vi "Bernards.vi"() -> ()   [LabVIEW 2018]
uses:
  <userlib>/KE237.LLB/Keith 237 Operate/Standby.vi
  <vilib>/Utility/file.llb/Write Delimited Spreadsheet (string).vi
  <instrlib>/Keithley 24XX/Keithley 24XX.lvlib
  <vilib>/Analysis/NI_AALBase.lvlib
panel:
  out "error 2":string
  out "error":string
  in  "Delay Gate (s) 2":dbl=60.0 format="%#.3g"
  in  "source/measure (V/I:0)":u16(ring)=1 items=["voltage/current", "current/voltage"]
  in  "Setpoint Array":dbl[](array[numeric])=[-2e-08, -5e-08, -1e-07]
  in  "Autozero?":u16(ring)=2 items=["On", "Off", "Once"]
  in  "Measurement Speed (1 PLC)":dbl=1.0 format="%.2g"
  in  "Manual Range (Max I)":dbl=1.0
  in  "Enable Meas Auto Range":bool=TRUE
  in  "Source Mode":u16(ring) items=["Voltage", "Current"]
  in  "Initial Gate Setting":dbl format="%#.3g"
  in  "Voltage Compliance Limit 237 (V)":dbl=-0.95 format="%#.3f"
  in  "Current Compliance\nLimit 237 (A)":fxp<+/-,64,32>=0.10000000009313226
  in  "Delay Gate (s)":dbl=30.0 format="%#.3g"
  in  "Keithley 237 GPIB address":string="17"
  in  "Wait Time Btwn Keithley Readings (ms)":i32=30
  out "Time Btwn Iterations (ms)":i32
  out "Total Elapsed Time (ms)":i32
  out "# Avgs":i32
  out "Current (A)":dbl format="%.2e"
  in  "Total Measure Time (s)":dbl=120.0 format="%#.3g"
  in  "Drain Bias (V)":dbl=-0.6 format="%#.3g"
  in  "Current Compliance\nLimit (A)":dbl=0.5 format="%#.3e"
  in  "Keithley 2400\nVISA resource":refnum<visa-resource-name>="GPIB0::24::INSTR"
  in  "ApproximateTime Step (ms)":dbl=300.0 format="%#.3g"
  in  "Current Offset":dbl format="%^#_3e"
  out "I-t Measurement\nBy M. Ziffer 7/3/2014":cluster{dbl[], dbl[]}(graph)={[-2.0, -1.95, -1.9, -1.85, -1.8, -1.75, -1.7, -1.65, -1.6, -1.55, -1.5, -1.45, -1.4, -1.35, -1.2999999999999998, -1.25, -1.2, -1.15, -1.1, -1.0499999999999998, -1.0, -0.95, -0.8999999999999999, -0.8499999999999999, -0.7999999999999998, -0.75, -0.7, -0.6499999999999999, -0.5999999999999999, -0.5499999999999998, -0.5, -0.44999999999999996, -0.3999999999999999, -0.34999999999999987, -0.2999999999999998, -0.25, -0.19999999999999996, -0.1499999999999999, -0.09999999999999987, -0.04999999999999982, 0.0, 0.050000000000000266, 0.10000000000000009, 0.1499999999999999, 0.20000000000000018, 0.25, 0.30000000000000027, 0.3500000000000001, 0.40000000000000036, 0.4500000000000002, 0.5, 0.5500000000000003, 0.6000000000000001, 0.6500000000000004, 0.7000000000000002, 0.75, 0.8000000000000003, 0.8500000000000001, 0.9000000000000004, 0.9500000000000002, 1.0, 1.0500000000000003, 1.1, 1.1500000000000004, 1.2000000000000002, 1.25, 1.3000000000000003, 1.35, 1.4000000000000004, 1.4500000000000002, 1.5, 1.5500000000000003, 1.6, 1.6500000000000004, 1.7000000000000002, 1.75, 1.8000000000000003, 1.85, 1.9000000000000004, 1.9500000000000002, 2.0, 1.95, 1.9, 1.85, 1.8, 1.75, 1.7, 1.65, 1.6, 1.55, 1.5, 1.45, 1.4, 1.35, 1.2999999999999998, 1.25, 1.2, 1.15, 1.1, 1.0499999999999998, 1.0, 0.95, 0.8999999999999999, 0.8499999999999999, 0.7999999999999998, 0.75, 0.7, 0.6499999999999999, 0.5999999999999999, 0.5499999999999998, 0.5, 0.44999999999999996, 0.3999999999999999, 0.34999999999999987, 0.2999999999999998, 0.25, 0.19999999999999996, 0.1499999999999999, 0.09999999999999987, 0.04999999999999982, 0.0, -0.050000000000000266, -0.10000000000000009, -0.1499999999999999, -0.20000000000000018, -0.25, -0.30000000000000027, -0.3500000000000001, -0.40000000000000036, -0.4500000000000002, -0.5, -0.5500000000000003, -0.6000000000000001, -0.6500000000000004, -0.7000000000000002, -0.75, -0.8000000000000003, -0.8500000000000001, -0.9000000000000004, -0.9500000000000002, -1.0, -1.0500000000000003, -1.1, -1.1500000000000004, -1.2000000000000002, -1.25, -1.3000000000000003, -1.35, -1.4000000000000004, -1.4500000000000002, -1.5, -1.5500000000000003, -1.6, -1.6500000000000004, -1.7000000000000002, -1.75, -1.8000000000000003, -1.85, -1.9000000000000004, -1.9500000000000002, -2.0], [-0.9617289445307117, -0.9618513744908972, -0.9601574911889584, -0.9603488957746004, -0.9598860982876659, -0.9595594700613103, -0.9590290885663679, -0.9586886097902229, -0.9580144940757807, -0.9570474587019399, -0.9571418538143588, -0.9562287187728303, -0.9551771894828052, -0.9535572870291384, -0.9535421571112963, -0.9533114258642045, -0.9520938012261039, -0.9513117179729429, -0.9508812384355169, -0.9504840780921618, -0.9504173840793213, -0.9482281628421478, -0.9464640811713977, -0.9453356785488072, -0.9439408336230415, -0.9428695575652444, -0.9416178906119992, -0.9396031084275935, -0.9378375248899987, -0.9354517815949719, -0.9324159524550173, -0.928767917889437, -0.9245502864168607, -0.9203528467096396, -0.9146985405384399, -0.908595454304189, -0.9012966039381313, -0.8917361646028689, -0.8808115851751085, -0.8684870433493713, -0.853007079283089, -0.8360736418594031, -0.8154860511533626, -0.7920970894092216, -0.7641180332150388, -0.7294003786125389, -0.6854183749419586, -0.6263231964633708, -0.5399961516707377, -0.4044042921440459, -0.19129744134883978, 0.11936942255465804, 0.5420583260977958, 1.0996962734707192, 1.8318907919106253, 2.7834859177196174, 3.9948214605959804, 5.494887344369723, 7.293988211209965, 9.39251059714275, 11.765998658717283, 14.371720946722268, 17.153138293174568, 20.070768287470067, 23.082285540692517, 26.15604905590766, 29.26009131920428, 32.38734131897913, 35.54092126952808, 38.70923397757575, 41.89103456238207, 45.09512285116253, 48.318234786641504, 51.57411300669423, 54.84161623237131, 58.130390342544004, 61.4596508891188, 64.79419021952893, 68.17503711098149, 71.57587551887687, 75.0023346626475, 71.8977923333163, 68.72637799211101, 65.51757272894447, 62.2950059155054, 59.076872390492845, 55.84672949319313, 52.615591470047114, 49.383497814590335, 46.15858586388574, 42.93308596012382, 39.714879010509975, 36.494540522470736, 33.276879251143754, 30.087779593472593, 26.903443634933772, 23.758388169345494, 20.669969771208738, 17.671195580039395, 14.804861569698371, 12.12778391916459, 9.68736655227705, 7.528128139792144, 5.673530623057721, 4.128839936603901, 2.8787577310032053, 1.895544581260216, 1.1383875896205915, 0.5622048852612092, 0.12746496878202787, -0.18928305409978952, -0.4042961076690051, -0.5411369085387429, -0.6286316214282486, -0.6871327837574404, -0.7298882072135505, -0.7640718647157413, -0.7921132761963248, -0.8155779431543743, -0.8358809022810104, -0.8523300154596555, -0.8668520109778625, -0.8802307520791266, -0.8907705198464766, -0.8998007445608903, -0.9078572589377096, -0.9150023626386364, -0.9215738644543149, -0.925261336930741, -0.9288795566582202, -0.9332418679701618, -0.9352489739462505, -0.9376688708058178, -0.9394550911063516, -0.9405290371496502, -0.9430050037047499, -0.9440335043698243, -0.9453382929096107, -0.9473152502994113, -0.9474565926568992, -0.9494901203645137, -0.94896546821346, -0.9503187058651598, -0.9511280452203158, -0.9523093469306558, -0.9532668704811476, -0.9541692143312739, -0.9545545822386634, -0.955485183435348, -0.9561708134622656, -0.956805602515258, -0.9577699122788996, -0.9578049002139094, -0.9580356870856992, -0.958780001168953, -0.9592832934359943, -0.9588639388381576, -0.959203916992021, -0.9603773199952523, -0.9611007191920772, -0.9623172869609168]}
  in  "First bias settle (ms)":dbl=2000.0 format="%#.2f"
  out "Outputfile":path
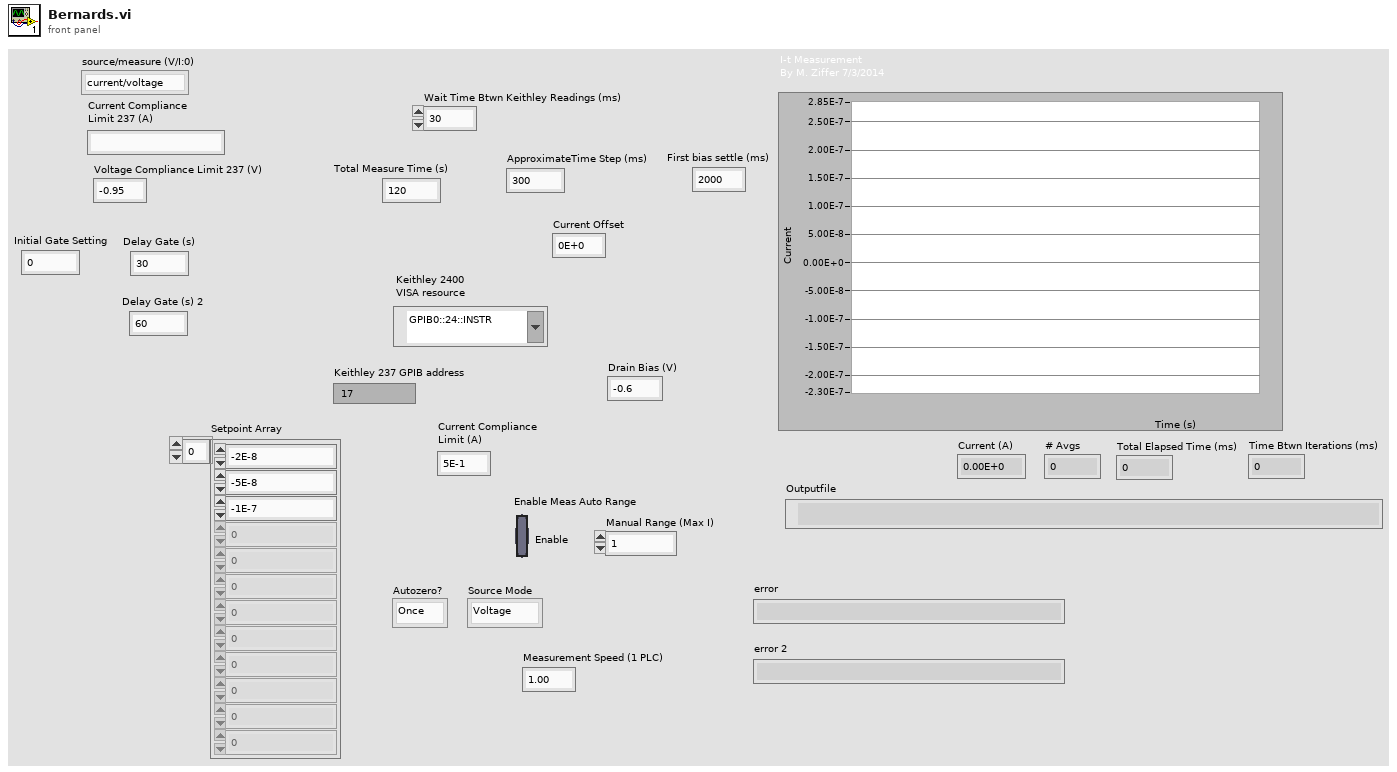
[diagram p1: front panel]
types:
  T1 = cluster{"error":bool, "code":i32, "source":string}
  T2 = cluster{"source value":string, "measure value":string, "delay value (sec)":string, "time value (sec)":string}[]
  T3 = cluster{"source value":dbl, "measure value":dbl, "delay value (sec)":dbl, "time value (sec)":dbl}[]
  T4 = cluster{"[0]":cluster{"source value":dbl, "measure value":dbl, "delay value (sec)":dbl, "time value (sec)":dbl}, "[1]":cluster{"source value":dbl, "measure value":dbl, "delay value (sec)":dbl, "time value (sec)":dbl}, "[2]":cluster{"source value":dbl, "measure value":dbl, "delay value (sec)":dbl, "time value (sec)":dbl}, "[3]":cluster{"source value":dbl, "measure value":dbl, "delay value (sec)":dbl, "time value (sec)":dbl}, "[4]":cluster{"source value":dbl, "measure value":dbl, "delay value (sec)":dbl, "time value (sec)":dbl}, "[5]":cluster{"source value":dbl, "measure value":dbl, "delay value (sec)":dbl, "time value (sec)":dbl}, "[6]":cluster{"source value":dbl, "measure value":dbl, "delay value (sec)":dbl, "time value (sec)":dbl}, "[7]":cluster{"source value":dbl, "measure value":dbl, "delay value (sec)":dbl, "time value (sec)":dbl}, "[8]":cluster{"source value":dbl, "measure value":dbl, "delay value (sec)":dbl, "time value (sec)":dbl}}
  T5 = cluster{"source value":dbl, "measure value":dbl, "delay value (sec)":dbl, "time value (sec)":dbl}
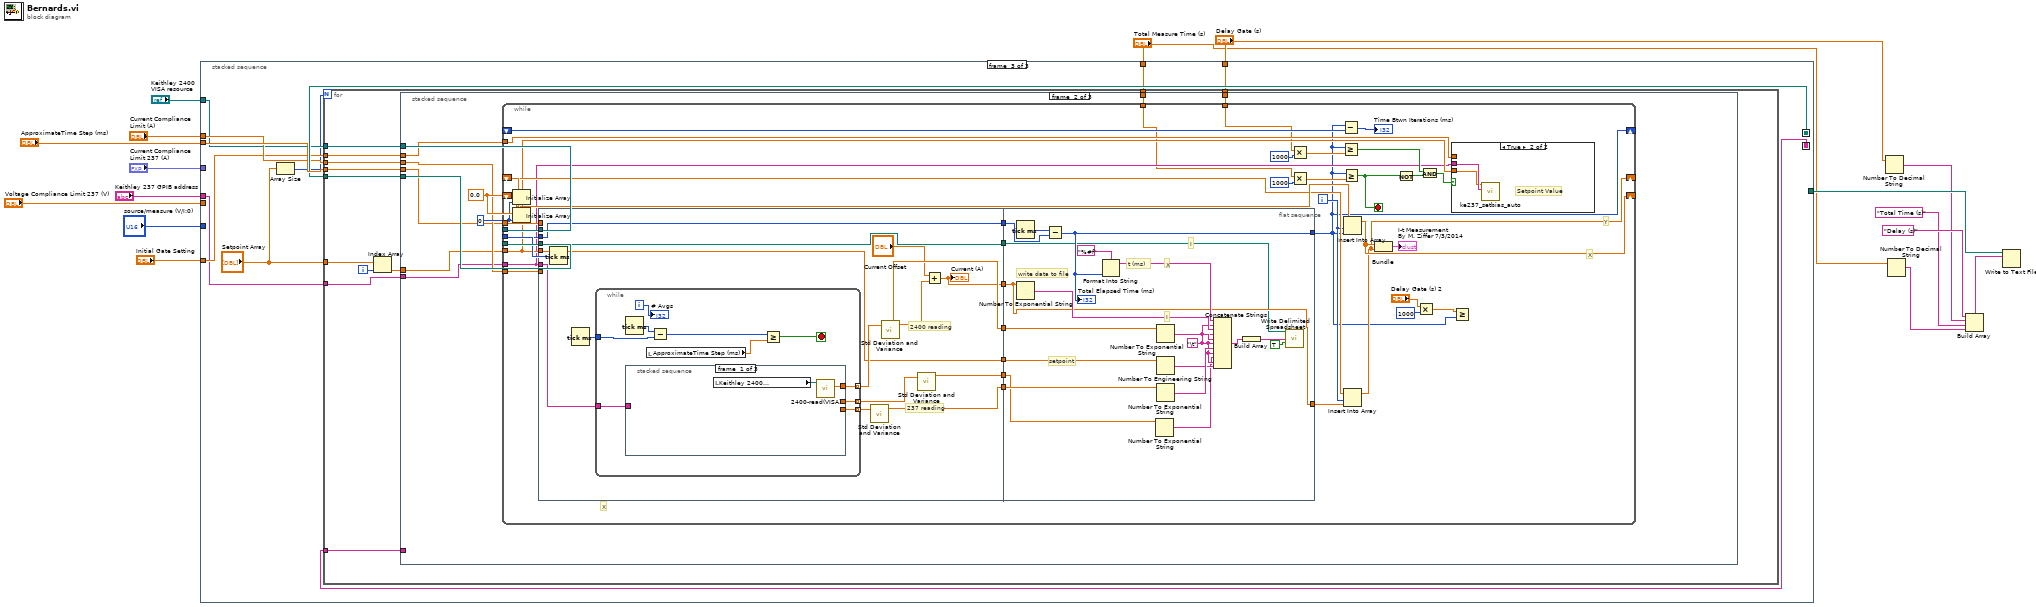
[diagram p0: block diagram]
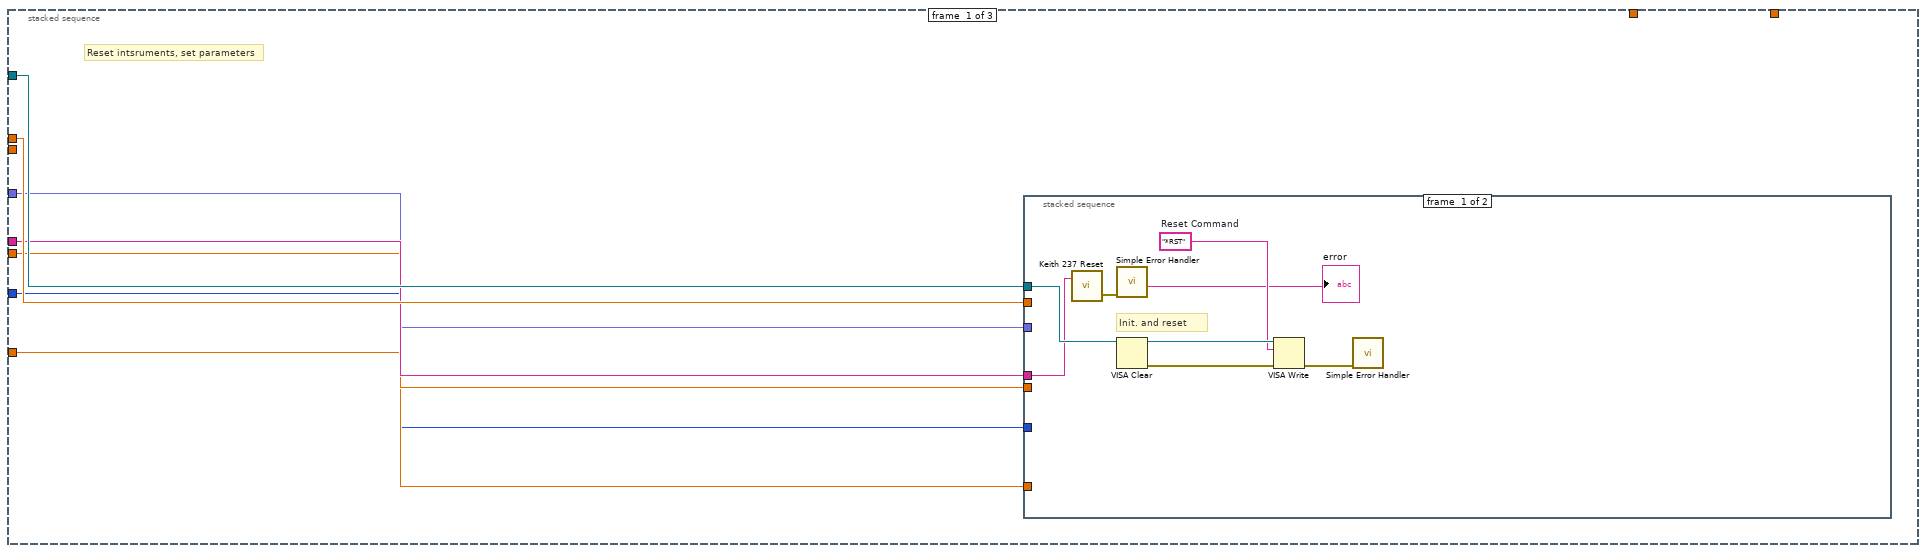
[diagram p2: hidden frame]
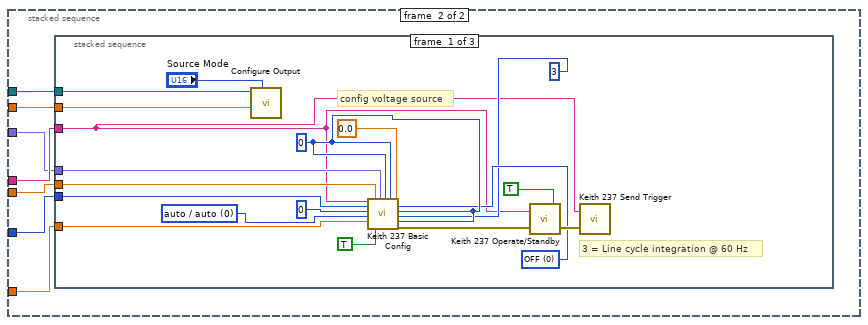
[diagram p3: hidden frame]
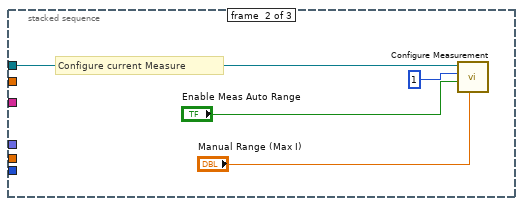
[diagram p4: hidden frame]
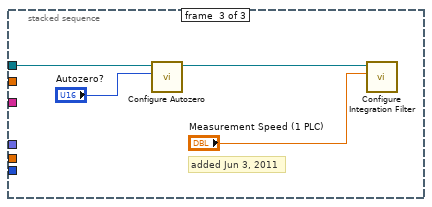
[diagram p5: hidden frame]
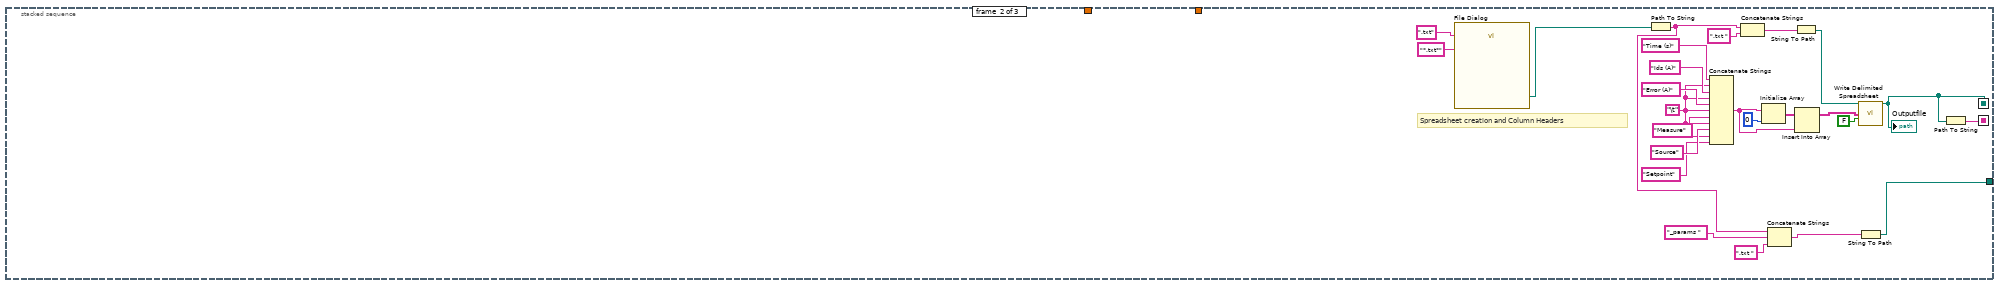
[diagram p6: hidden frame]
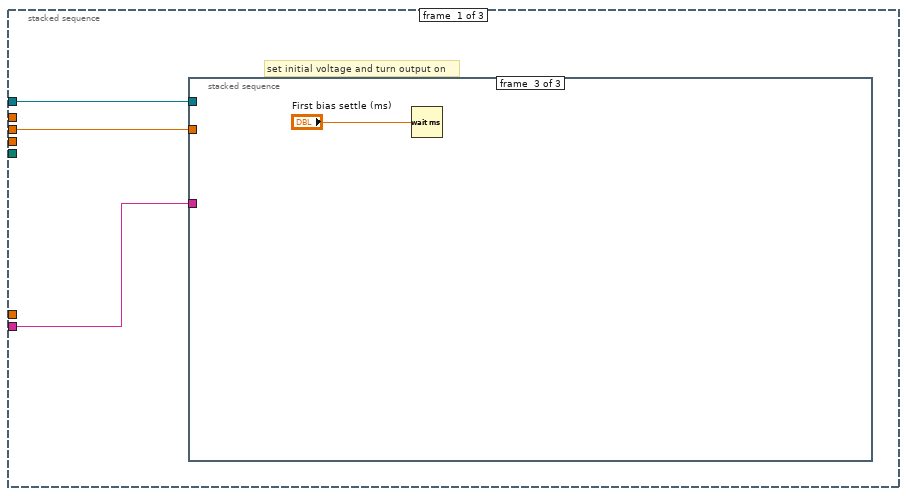
[diagram p7: hidden frame]
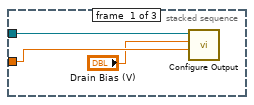
[diagram p8: hidden frame]
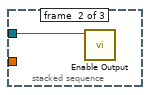
[diagram p9: hidden frame]
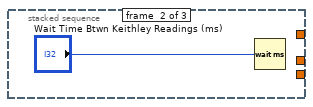
[diagram p10: hidden frame]
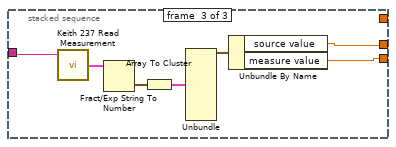
[diagram p11: hidden frame]
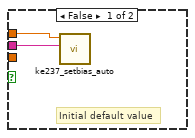
[diagram p12: hidden frame]
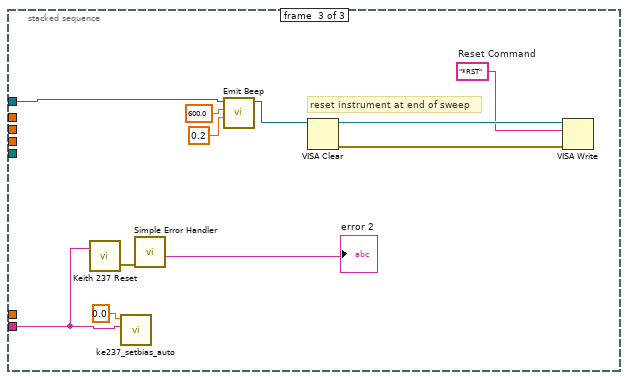
[diagram p13: hidden frame]
diagram:
  n1 = stacked-sequence {
    seq-local: [_ w70 _] -> [_ _ w99]
    seq-local: [_ w89 _] -> [_ _ w98]
    tunnel: "ApproximateTime Step (ms)" -> [_ _ w100]
    tunnel: "Keithley 2400\nVISA resource" -> [w22 _ w96]
    tunnel: "Current Compliance\nLimit (A)" -> [w23 _ w97]
    tunnel: "Keithley 237 GPIB address" -> [w21 _ w94]
    tunnel: "Voltage Compliance Limit 237 (V)" -> [w19 _ _]
    tunnel: "Current Compliance\nLimit 237 (A)" -> [w20 _ _]
    tunnel: "Initial Gate Setting" -> [w18 _ w95]
    tunnel: "source/measure (V/I:0)" -> [w17 _ _]
    tunnel: [_ w65 _] -> w6
    tunnel: "Delay Gate (s)" -> [_ _ w91]
    tunnel: "Total Measure Time (s)" -> [_ _ w90]
    frame #0 {
      # "Reset intsruments, set parameters"
      n2 = stacked-sequence {
        tunnel: w22 -> [w31 w37]
        tunnel: w23 -> [_ w38]
        tunnel: w21 -> [w25 w36]
        tunnel: w20 -> [_ w35]
        tunnel: w19 -> [_ w34]
        tunnel: w18 -> [_ w33]
        tunnel: w17 -> [_ w32]
        frame #0 {
          w29 = "*RST"  # Reset Command
          # "Init. and reset"
          n3 = call <userlib>:"Keith 237 Reset.vi"("GPIB address"=w25) -> ("error out"=w26:T1)  [unwired: 1 in]
          n4 = call <vilib>:"Simple Error Handler.vi"("error in (no error)"=w26) -> ("source out"=→"error":string)  [unwired: 1 in, 7 out]
          n5 = VISA Clear(VISA resource name=w31) -> (VISA resource name out=w30:refnum<visa-resource-name>, error out=w28:errorcluster)  [unwired: 1 in]
          n6 = VISA Write(VISA resource name=w30, write buffer=w29, error in (no error)=w28) -> (error out=w27:errorcluster)  [unwired: 2 out]
          n7 = call <vilib>:"Simple Error Handler.vi"("error in (no error)"=w27) -> ()  [unwired: 1 in, 8 out]
        }
        frame #1 {
          n8 = stacked-sequence {
            tunnel: w37 -> [w56 w59 w63]
            tunnel: w38 -> [w55 _ _]
            tunnel: w36 -> [w40 _ _]
            tunnel: w35 -> [w43 _ _]
            tunnel: w34 -> [w42 _ _]
            tunnel: w33 -> [w41 _ _]
            tunnel: w32 -> [w39 _ _]
            frame #0 {
              w45 = u16 0 items=["OFF", "ON"] ("default delay (on:1)")
              w46 = u16 0 items=["auto / auto", "1 nA / 1.1 V", "10 nA / 11 V", "100 nA / 110 V", "0.001 mA / 1100 V", "0.01 mA / 1100 V", "0.1 mA / 1100 V", "1 mA / 1100 V", "10 mA / 1100 V", "100 mA / 1100 V"] ("source range\nI source / V source (auto:0)")
              w48 = u16 0
              # "3 = Line cycle integration @ 60 Hz"
              # "config voltage source"
              n9 = call <instrlib>:"Configure Output.vi"("Source Mode  (0: Voltage)"="Source Mode", "Compliance  Level (0.1)"=w55, "VISA resource name"=w56) -> ()  [unwired: 3 in, 6 out]
              n10 = call <userlib>:"Keith 237 Basic Config.vi"("GPIB address"=w40, "source/measure (V/I:0)"=w39, "function (DC:0)"=u16 0, "source range\nI source / V source (auto:0)"=w46, "source level"=w41, "voltage \ncompliance level"=w42, "1100 V range (disabled:F)"=TRUE, "current \ncompliance level"=w43, "compliance/\nmeasurement range (auto:0)"=w48, "suppression (off:0)"=w48, "DC delay (sec)"=0.0, "default delay (on:1)"=w45, "filter (disabled:0)"=w48, "integration time (medium:1)"=u16 3, "sense (local:0)"=w48) -> ("error out"=w53:T1)  [unwired: 4 in]
              n11 = call "Keith 237 Operate/Standby.vi"("source"=TRUE, "error in"=w53, "GPIB address"=w40) -> ("error out"=w51:T1)
              n12 = call <userlib>:"Keith 237 Send Trigger.vi"("GPIB address"=w40, "error in"=w51) -> ()  [unwired: 1 out]
            }
            frame #1 {
              # "Configure current Measure"
              n13 = call <instrlib>:"Configure Measurement.vi"("Manual Range (1.0)"="Manual Range (Max I)", "Enable Auto Range (T:Enable)"="Enable Meas Auto Range", "Function (0: Volts)"=1, "VISA resource name"=w59) -> ()  [unwired: 1 in, 7 out]
            }
            frame #2 {
              # "added Jun 3, 2011"
              n14 = call <instrlib>:"Configure Autozero.vi"("Autozero  (0: On)"="Autozero?", "VISA resource name"=w63) -> ("VISA resource name out"=w62:refnum<visa-resource-name>)  [unwired: 1 in, 8 out]
              n15 = call <instrlib>:"Configure Integration Filter.vi"("Measurement Speed (1 PLC)"="Measurement Speed (1 PLC)", "VISA resource name"=w62) -> ()  [unwired: 8 in, 2 out]
            }
          }
        }
      }
    }
    frame #1 {
      w72 = "\t"
      # "Spreadsheet creation and Column Headers"
      n16 = call "File Dialog"("default name"=".txt", "pattern (all files)"="*.txt*") -> ("selected path"=w76:path)  [unwired: 5 in, 8 out]
      n17 = Path To String(path=w76) -> (string=w67:string)
      n18 = Concatenate Strings("Time (s)", w72, "Ids (A)", w72, "Error (A)", w72, "Measure", w72, "Source", w72, "Setpoint") -> (w87:string)
      n19 = Concatenate Strings(w67, ".txt " ("string")) -> (w75:string)
      n20 = Initialize Array(w87, 0 ("dimension size")) -> (w86:string[])
      n21 = Concatenate Strings(w67, "_params " ("string"), ".txt " ("string")) -> (w66:string)
      n22 = String To Path(string=w75) -> (path=w74:path)
      n23 = Insert Into Array(array=w86, new element=w87) -> (w79:string[])  [unwired: 1 in]
      n24 = call-poly <vilib>:"Write Delimited Spreadsheet.vi"("file path (dialog if empty)"=w74, "1D data"=w79, "append to file? (new file:F)"=FALSE) -> ("new file path (Not A Path if cancelled)"=w70:path)  [unwired: 11 in, 1 out]
      "Outputfile" <- w70
      n25 = String To Path(string=w66) -> (path=w65:path)
      n26 = Path To String(path=w70) -> (string=w89:string)
    }
    frame #2 {
      n27 = Array Size(array="Setpoint Array") -> (size(s)=w92:i32)
      n28 = for {
        N: w92 -> [_]
        tunnel: w100 -> [w112]
        tunnel: w99 -> [w111]
        tunnel: w98 -> [w110]
        tunnel: w97 -> [w109]
        tunnel: w96 -> [w108]
        tunnel: w95 -> [w107]
        tunnel: w94 -> [w101]
        tunnel: "Setpoint Array" -> [w106]
        tunnel: w91 -> [w103]
        tunnel: w90 -> [w102]
        i -> [w104]
        n29 = Index Array(array=w106, index=w104) -> (element=w105:dbl)
        n30 = stacked-sequence {
          tunnel: w112 -> [_ w127 _]
          tunnel: w111 -> [_ w134 _]
          tunnel: w110 -> [_ _ _]
          tunnel: w109 -> [w115 w128 _]
          tunnel: w108 -> [w114 w129 w238]
          tunnel: w107 -> [_ w125 _]
          tunnel: w101 -> [w113 w121 w232]
          tunnel: w105 -> [_ w124 _]
          tunnel: w103 -> [_ w123 _]
          tunnel: w102 -> [_ w122 _]
          frame #0 {
            # "set initial voltage and turn output on"
            n31 = stacked-sequence {
              tunnel: w114 -> [w117 w119 _]
              tunnel: w115 -> [w118 _ _]
              tunnel: w113 -> [_ _ _]
              frame #0 {
                n32 = call <instrlib>:"Configure Output.vi"("Compliance  Level (0.1)"=w118, "Output Level (0)"="Drain Bias (V)", "VISA resource name"=w117) -> ()  [unwired: 3 in, 6 out]
              }
              frame #1 {
                n33 = call <instrlib>:"Enable Output.vi"("VISA resource name"=w119) -> ()  [unwired: 2 in, 9 out]
              }
              frame #2 {
                n34 = Wait (ms)(milliseconds to wait="First bias settle (ms)") -> ()  [unwired: 1 out]
              }
            }
          }
          frame #1 {
            w130 = 0
            w131 = 0.0
            n35 = Initialize Array(w131, w130) -> (w132:dbl[])
            n36 = Initialize Array(w131, w130) -> (w133:dbl[])
            n37 = Tick Count (ms)() -> (millisecond timer value=w126:u32)
            n38 = while {
              shift-left: w132 -> [w169]
              shift-right: [w164] -> _
              shift-left: w133 -> [w170]
              shift-right: [w166] -> _
              tunnel: w134 -> [w171]
              tunnel: w129 -> [w168]
              tunnel: w128 -> [w167]
              tunnel: w127 -> [w162]
              tunnel: w126 -> [w157]
              shift-right: [w139] -> _
              shift-left: _ -> [w161]
              tunnel: w121 -> [w148]
              tunnel: w125 -> [w154]
              tunnel: w124 -> [w149]
              tunnel: w123 -> [w136]
              tunnel: w122 -> [w135]
              i -> [w163]
              stop <- w153 stop-if-true
              # "X"
              # "X"
              # "Y"
              n39 = flat-sequence {
                tunnel: w171 -> [w178]
                tunnel: [w178] -> w147
                tunnel: w168 -> [_]
                tunnel: w167 -> [_]
                tunnel: w162 -> [_]
                tunnel: w157 -> [w177]
                tunnel: [w177] -> w146
                tunnel: w149 -> [w176]
                tunnel: [w176] -> w145
                tunnel: w148 -> [w180]
                tunnel: [w185] -> w144
                tunnel: [w181] -> w143
                tunnel: [w175] -> w142
                tunnel: [w173] -> w137
                tunnel: [w212] -> w165
                tunnel: w147 -> [w207]
                tunnel: w146 -> [w219]
                tunnel: [w218] -> w139
                tunnel: w145 -> [w215]
                tunnel: w144 -> [w221]
                tunnel: w143 -> [w212]
                tunnel: w142 -> [w214]
                tunnel: w137 -> [w208]
                frame #0 {
                  # "2400 reading"
                  # "237 reading"
                  n40 = Tick Count (ms)() -> (millisecond timer value=w182:u32)
                  n41 = while {
                    tunnel: [w196] -> w186 mode=indexing
                    tunnel: w182 -> [w194]
                    tunnel: w180 -> [w189]
                    tunnel: [w188] -> w179 mode=indexing
                    tunnel: [w187] -> w174 mode=indexing
                    i -> [w195]
                    stop <- w192 stop-if-true
                    n42 = Tick Count (ms)() -> (millisecond timer value=w191:u32)
                    n43 = stacked-sequence {
                      tunnel: [w197 _ _] -> w196
                      tunnel: w189 -> [_ _ w202]
                      tunnel: [_ _ w200] -> w188
                      tunnel: [_ _ w201] -> w187
                      frame #0 {
                        n44 = local read "Keithley 2400\nVISA resource"() -> (w198:refnum<visa-resource-name>)
                        n45 = call "2400-read(VISA).vi"("2400 VISA ID"=w198) -> ("Current"=w197:dbl)  [unwired: 6 out]
                      }
                      frame #1 {
                        n46 = Wait (ms)(milliseconds to wait="Wait Time Btwn Keithley Readings (ms)") -> ()  [unwired: 1 out]
                      }
                      frame #2 {
                        n47 = call <userlib>:"Keith 237 Read Measurement.vi"("GPIB address"=w202) -> ("display"=w204:T2)  [unwired: 1 in, 3 out]
                        n48 = Fract/Exp String To Number(string=w204) -> (number=w205:T3)  [unwired: 3 in, 1 out]
                        n49 = Array To Cluster(array=w205) -> (cluster=w206:T4)
                        n50 = Unbundle(w206) -> ("[0]"=w203:T5)  [unwired: 8 out]
                        n51 = Unbundle By Name(w203) -> ("source value"=w201:dbl, "measure value"=w200:dbl)
                      }
                    }
                    n52 = local read "ApproximateTime Step (ms)"() -> (w190:dbl)
                    n53 = Subtract(x=w191, y=w194) -> (x-y=w193:u32)
                    n54 = Greater Or Equal?(x=w193, y=w190) -> (x >= y?=w192:bool)
                    "# Avgs" <- w195
                  }
                  n55 = call <vilib>:"Std Deviation and Variance.vi"("X"=w179) -> ("mean"=w175:dbl)  [unwired: 1 in, 2 out]
                  n56 = call <vilib>:"Std Deviation and Variance.vi"("X"=w186) -> ("mean"=w184:dbl, "standard deviation"=w185:dbl)  [unwired: 1 in, 1 out]
                  n57 = call <vilib>:"Std Deviation and Variance.vi"("X"=w174) -> ("mean"=w173:dbl)  [unwired: 1 in, 2 out]
                  n58 = Add(x="Current Offset", y=w184) -> (x+y=w181:dbl)
                  "Current (A)" <- w181
                }
                frame #1 {
                  w210 = "\t"
                  # "setpoint"
                  # "I"
                  # "I"
                  # "t (ms)"
                  # "write data to file"
                  # "X"
                  n59 = Tick Count (ms)() -> (millisecond timer value=w220:u32)
                  n60 = Number To Exponential String(number=w212) -> (E-format string=w224:string)  [unwired: 3 out]
                  n61 = Subtract(x=w220, y=w219) -> (x-y=w218:u32)
                  "Total Elapsed Time (ms)" <- w218
                  n62 = Format Into String(format string="%#f", w218) -> (resulting string=w225:string)  [unwired: 2 in, 1 out]
                  n63 = Number To Exponential String(number=w208) -> (E-format string=w209:string)  [unwired: 3 out]
                  n64 = Number To Exponential String(number=w221) -> (E-format string=w222:string)  [unwired: 3 out]
                  n65 = Number To Engineering String(4:w215) -> (0:w211:string)  [unwired: 3 in]
                  n66 = Number To Exponential String(number=w214) -> (E-format string=w213:string)  [unwired: 3 out]
                  n67 = Concatenate Strings(w225, w210, w224, w210, w222, w210, w213, w210, w209, w210, w211) -> (w223:string)
                  n68 = Build Array(w223) -> (w217:string[])
                  n69 = call-poly <vilib>:"Write Delimited Spreadsheet.vi"("file path (dialog if empty)"=w207, "1D data"=w217, "append to file? (new file:F)"=TRUE) -> ()  [unwired: 11 in, 2 out]
                }
              }
              n70 = Multiply(x=w136, y=1000) -> (x*y=w156:dbl)
              n71 = Multiply(x=w135, y=1000) -> (x*y=w158:dbl)
              n72 = Subtract(x=w139, y=w161) -> (x-y=→"Time Btwn Iterations (ms)":u32)
              n73 = Greater Or Equal?(x=w139, y=w156) -> (x >= y?=w151:bool)
              n74 = Greater Or Equal?(x=w139, y=w158) -> (x >= y?=w153:bool)
              n75 = Insert Into Array(array=w170, index=w163, new element=w139) -> (w166:dbl[])
              n76 = Insert Into Array(array=w169, index=w163, new element=w165) -> (w164:dbl[])
              n77 = Bundle(w166, w164) -> (→"I-t Measurement\nBy M. Ziffer 7/3/2014":cluster{dbl[], dbl[]})  [unwired: 1 out]
              n78 = Not(x=w153) -> (.not. x?=w152:bool)
              n79 = Multiply(x="Delay Gate (s) 2", y=1000) -> (x*y=w138:dbl)
              n80 = And(x=w151, y=w152) -> (x .and. y?=w150:bool)
              n81 = case shown="True" w150 {
                tunnel: w148 -> [w228 w230]
                tunnel: w154 -> [w227 _]
                tunnel: w149 -> [_ w229]
                frame False {
                  # "Initial default value"
                  n82 = call "ke237_setbias_auto.vi"("GPIB address"=w228, "source level"=w227) -> ()  [unwired: 10 in]
                }
                frame True {
                  # "Setpoint Value"
                  n83 = call "ke237_setbias_auto.vi"("GPIB address"=w230, "source level"=w229) -> ()  [unwired: 10 in]
                }
              }
              n84 = Greater Or Equal?(x=w138, y=w139) -> ()  [unwired: 1 out]
            }
          }
          frame #2 {
            w240 = "*RST"  # Reset Command
            # "reset instrument at end of sweep"
            n85 = call <userlib>:"Keith 237 Reset.vi"("GPIB address"=w232) -> ("error out"=w233:T1)  [unwired: 1 in]
            n86 = call "ke237_setbias_auto.vi"("GPIB address"=w232, "source level"=0.0) -> ()  [unwired: 10 in]
            n87 = call <vilib>:"Simple Error Handler.vi"("error in (no error)"=w233) -> ("source out"=→"error 2":string)  [unwired: 1 in, 7 out]
            n88 = call <instrlib>:"Emit Beep.vi"("Beep Duration (.25 s)"=0.2, "Beep Frequency (300)"=600.0, "VISA resource name"=w238) -> ("VISA resource name out"=w237:refnum<visa-resource-name>)  [unwired: 7 in, 1 out]
            n89 = VISA Clear(VISA resource name=w237) -> (VISA resource name out=w241:refnum<visa-resource-name>, error out=w239:errorcluster)  [unwired: 1 in]
            n90 = VISA Write(VISA resource name=w241, write buffer=w240, error in (no error)=w239) -> ()  [unwired: 3 out]
          }
        }
      }
    }
  }
  n91 = Number To Decimal String(number="Delay Gate (s)") -> (decimal integer string=w5:string)  [unwired: 1 in]
  n92 = Number To Decimal String(number="Total Measure Time (s)") -> (decimal integer string=w2:string)  [unwired: 1 in]
  n93 = Build Array("Delay (s)", w5, "Total Time (s)", w2) -> (w8:string[])
  n94 = Write to Text File(file (use dialog)=w6, text=w8) -> ()  [unwired: 2 in, 3 out]
